vi "AMI model value.vi"(1 "AMI Model":enum16{"MODEL 420", "MODEL 430"}(ring), 2 "Read/Write this vi":bool) -> (0 "AMI Model 2":enum16{"MODEL 420", "MODEL 430"}(ring))   [LabVIEW 2021]
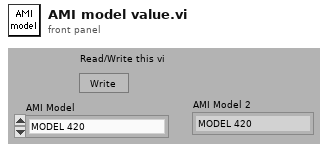
[diagram p1: front panel]
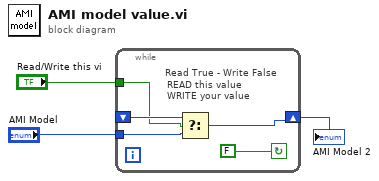
[diagram p0: block diagram]
diagram:
  n1 = while {
    shift-right: [w7] -> w2
    shift-left: _ -> [w6]
    tunnel: "Read/Write this vi" -> [w4]
    tunnel: "AMI Model" -> [w8]
    stop <- FALSE continue-if-true
    # "READ this value\nWRITE your value"
    # "Read True - Write False"
    n2 = Select(t=w6, s=w4, f=w8) -> (s? t:f=w7:enum16{"MODEL 420", "MODEL 430"})
  }
  "AMI Model 2" <- w2
